vi "AVS_SetAnalogOut.vi"(0 "a_hDevice":i32, 7 "a_PortId":u8, 11 "a_Value":sgl) -> (4 "Output Value":i32)   [LabVIEW 2016]
uses:
  libavs.so
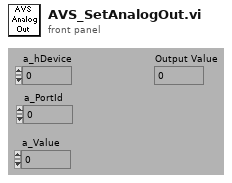
[diagram p1: front panel]
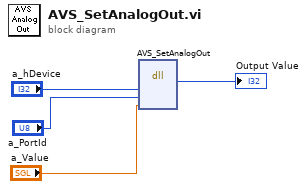
[diagram p0: block diagram]
diagram:
  n1 = dll-call lib="home/harini/tcs/ts_sedspectrometer/ss_sedspectrometer/VIs/libavs.so" fn="AVS_SetAnalogOut"("a_hDevice"="a_hDevice", "a_PortId"="a_PortId", "a_Value"="a_Value") -> ("return type"=→"Output Value":i32)  [unwired: 6 in, 2 out]
